vi "HD_name_to_IP_No_mapper.vi"(1 "Mode":T1(ring), 2 "Input":string) -> (0 "Output":string)   [LabVIEW 2010]
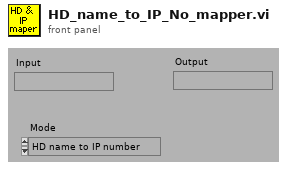
[diagram p1: front panel]
types:
  T1 = enum16{"HD name to IP number", "IP number to HD name"}
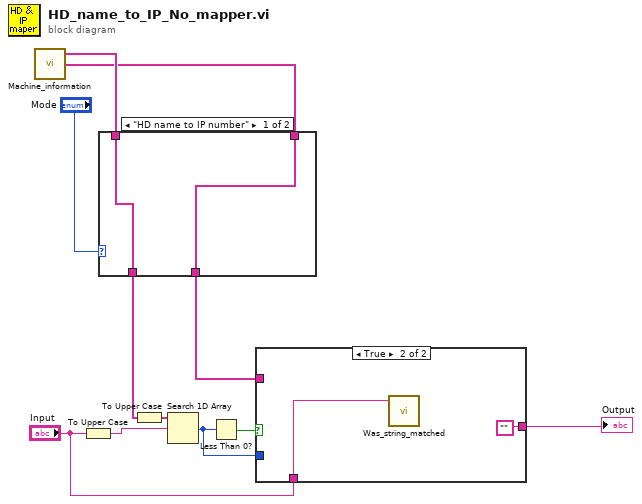
[diagram p0: block diagram]
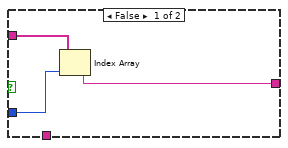
[diagram p2: hidden frame]
diagram:
  n1 = call "Machine_information.vi"() -> ("Machine:IP:Number"=w1:string[], "Machine:HD:Name"=w2:string[])  [unwired: 1 in]
  n2 = To Upper Case(1:"Input") -> (0:w4:string)
  n3 = case shown="\"HD name to IP number\"" "Mode" {
    tunnel: [w13 w15] -> w10
    tunnel: w2 -> [w13 w14]
    tunnel: w1 -> [w12 w15]
    tunnel: [w12 w14] -> w6
    frame "HD name to IP number" {
    }
    frame "IP number to HD name" {
    }
  }
  n4 = To Upper Case(1:w10) -> (0:w5:string[])
  n5 = Search 1D Array(1D array=w5, element=w4) -> (index of element=w7:i32)  [unwired: 1 in]
  n6 = Less Than 0?(x=w7) -> (x < 0?=w9:bool)
  n7 = case shown="True" w9 {
    tunnel: [w16 ""] -> w8
    tunnel: w7 -> [w18 _]
    tunnel: w6 -> [w17 _]
    tunnel: "Input" -> [_ w20]
    frame False {
      n8 = Index Array(array=w17, index=w18) -> (element=w16:string)
    }
    frame True {
      n9 = call "Was_string_matched.vi"("Variable name"=w20) -> ()  [unwired: 2 in]
    }
  }
  "Output" <- w8
